vi "U8arrayToMeasurement.vi"(2 "factor 2":dbl=1000.0 format="%#_13g", 3 "factor 1":dbl=1000.0 format="%#_13g", 4 "payload":u8[](array[numeric])) -> (0 "Meas 2":dbl, 1 "Meas 1":dbl)   [LabVIEW 2021]
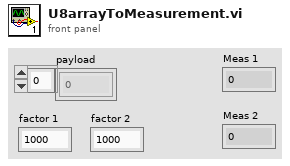
[diagram p1: front panel]
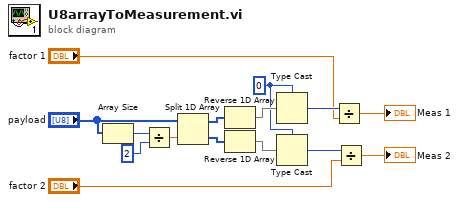
[diagram p0: block diagram]
diagram:
  w6 = 0
  n1 = Array Size(array="payload") -> (size(s)=w8:i32)
  n2 = Divide(x=w8, y=2) -> (x/y=w10:dbl)
  n3 = Split 1D Array(array="payload", index=w10) -> (first subarray=w11:u8[], second subarray=w12:u8[])
  n4 = Reverse 1D Array(array=w11) -> (reversed array=w13:u8[])
  n5 = Reverse 1D Array(array=w12) -> (reversed array=w14:u8[])
  n6 = Type Cast(type=w6, x=w13) -> (*(type *) &x=w15:i32)
  n7 = Type Cast(type=w6, x=w14) -> (*(type *) &x=w5:i32)
  n8 = Divide(x=w15, y="factor 1") -> (x/y=→"Meas 1":dbl)
  n9 = Divide(x=w5, y="factor 2") -> (x/y=→"Meas 2":dbl)
